vi "Read Temperature.vi"(8 "error in (no error)":errorcluster) -> (0 "error out":errorcluster)   [LabVIEW 2016]
uses:
  PPMS Global.vi
  instrument.PPMS2/instrument.PPMS2/instrument.PPMS2.lvclass
panel:
  out "Temperature (K)":dbl=299.9998
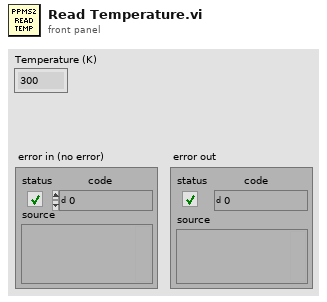
[diagram p1: front panel]
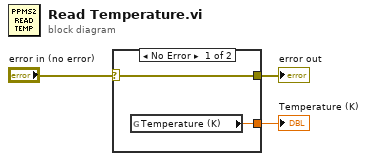
[diagram p0: block diagram]
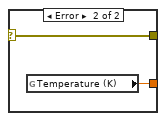
[diagram p2: hidden frame]
diagram:
  n1 = case shown="No Error" "error in (no error)" {
    selector: "error in (no error)" -> [w5 w7]
    tunnel: [w5 w7] -> w2
    tunnel: [w4 w6] -> w1
    frame No Error {
      n2 = global read "PPMS Global.vi" "Temperature (K)"() -> (w4:dbl)
    }
    frame Error {
      n3 = global read "PPMS Global.vi" "Temperature (K)"() -> (w6:dbl)
    }
  }
  "error out" <- w2
  "Temperature (K)" <- w1
